vi "Error.vi"(8 "error in":errorcluster, 10 "data":variant) -> (0 "error out":errorcluster)   [LabVIEW 2018, in "Display.lvlib"]
doc: "This VI enqueues the named action"
uses:
  Display.lvlib
  Private Controls/Module Data Cluster.ctl
  Private Controls/Module Action.ctl
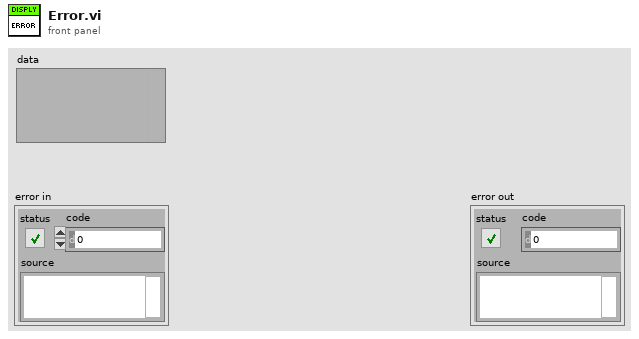
[diagram p1: front panel]
types:
  T1 = typedef "Display.lvlib/Module Data Cluster.ctl" = cluster{"Variant":variant, "action":T2}
  T2 = typedef "Display.lvlib/Module Action.ctl" = enum16{"error", "exit", "init", "Update Display"}
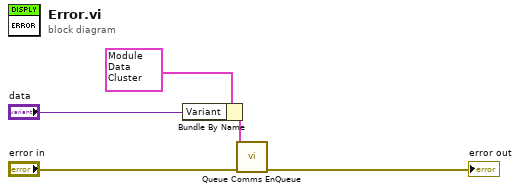
[diagram p0: block diagram]
diagram:
  n1 = Bundle By Name(cluster=T1 {"Variant"=variant, "action"=enum."error"} ("Module Data Cluster"), "Variant"="data") -> (w4:T1)
  n2 = call "Queue Comms EnQueue.vi"("error in"="error in", "Module Data Cluster"=w4) -> ("error out"=→"error out":errorcluster)  [unwired: 9 in]
